vi "Cleanup.vi"(8 "error in (no error)":errorcluster, 11 "ControlBindingPanel in":refnum<class "ControlBindingPanel.lvclass">) -> (0 "error out":errorcluster)   [LabVIEW 2020, in "VolatusGUIEditor.lvlib" / "ControlBindingPanel.lvclass"]
uses:
  ControlBindingPanel.lvclass
  ControlBindingPanel.lvclass/ControlBindingPanel.ctl
  lv-oopanel/OOPanel/Panel/Panel.lvclass
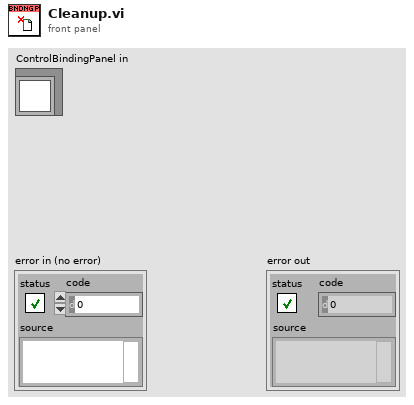
[diagram p1: front panel]
types:
  T1 = typedef "VolatusGUIEditor.lvlib/ControlBindingPanel.lvclass/Incoming Events.ctl" = cluster{"Update Control":refnum<user-event>, "Update Tree":refnum<user-event>}
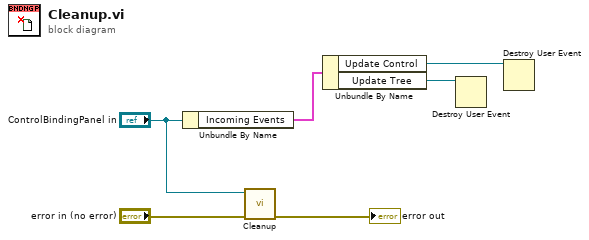
[diagram p0: block diagram]
diagram:
  n1 = Unbundle By Name("ControlBindingPanel in") -> ("Incoming Events"=w3:T1)
  n2 = call-parent "Cleanup.vi"("error in (no error)"="error in (no error)", "Panel in"="ControlBindingPanel in") -> ("error out"=→"error out":errorcluster)  [unwired: 9 in]
  n3 = Unbundle By Name(w3) -> ("Update Control"=w1:refnum<user-event>, "Update Tree"=w2:refnum<user-event>)
  n4 = Destroy User Event(user event=w2) -> ()  [unwired: 1 in, 1 out]
  n5 = Destroy User Event(user event=w1) -> ()  [unwired: 1 in, 1 out]
